vi "C(T) data viewer.vi"(0 "Cap Estimates":dbl[](array[numeric])=[1.269612045289484e-08, 1.3697308669126022e-08, 1.399985901178697e-08, 1.3777895246644411e-08, 1.3379717594157467e-08, 1.2501459178740452e-08, 1.1791524271713885e-08] format="%.2f", 1 "Temps":dbl[](array[numeric])=[26.0, 30.0, 34.0, 38.0, 42.0, 46.0, 50.0] format="%.2f", 2 "N Temps":i32=7, 5 "Resistance (Ohms)":dbl=100000.0 format="%.4e", 7 "Timing Control Parameters":T1={"N cycles for averaging"=300, "N points per measurement"=1000, "Measurment time interval"=2e-05} {"Measurment time interval" format="%.2e"}, 9 "waveforms":waveform(dbl)[](array[waveform])=[{"t0"=timestamp(3087922235.213 s since 1904-01-01), "dt"=1.9999999494757503e-05, "Y"=array[1000 elements]}, {"t0"=timestamp(3087922405.147 s since 1904-01-01), "dt"=1.9999999494757503e-05, "Y"=array[1000 elements]}, {"t0"=timestamp(3087922549.515 s since 1904-01-01), "dt"=1.9999999494757503e-05, "Y"=array[1000 elements]}, {"t0"=timestamp(3087922690.9379997 s since 1904-01-01), "dt"=1.9999999494757503e-05, "Y"=array[1000 elements]}, {"t0"=timestamp(3087922829.417 s since 1904-01-01), "dt"=1.9999999494757503e-05, "Y"=array[1000 elements]}, {"t0"=timestamp(3087922967.796 s since 1904-01-01), "dt"=1.9999999494757503e-05, "Y"=array[1000 elements]}, {"t0"=timestamp(3087923101.799 s since 1904-01-01), "dt"=1.9999999494757503e-05, "Y"=array[1000 elements]}], 11 "error in":errorcluster) -> (13 "no save out":bool, 15 "error out":errorcluster)   [LabVIEW 2016]
doc: "This vi allows the user to inspect the data before choosing to save it or not\n\nPaul K Dixon\nPhysics 350\nCSUSB Physics"
uses:
  globals/C(T) global variables.vi
panel:
  in  "Proceed no save":bool
  out "Resistance (Ohms)":dbl=100000.0 format="%.4e"
  out "Timing Control Parameters":T1={"N cycles for averaging"=300, "N points per measurement"=1000, "Measurment time interval"=2e-05} {"Measurment time interval" format="%.2e"}
  out "Number of Temperatures":i32=7
  out "Waveform":waveform(dbl)={"t0"=timestamp(3087922235.213 s since 1904-01-01), "dt"=1.9999999494757503e-05, "Y"=array[1000 elements]}
  out "Estimated Capacitance Value [nF]":i32(listbox) caption="choose the next state"
  out "Normalized decay versus time":waveform(dbl)(graph)={"t0"=timestamp(3087922235.213 s since 1904-01-01), "dt"=1.9999999494757503e-05, "Y"=array[1000 elements]}
  out "Cap versus Temp":cluster{"Temps":dbl[], dbl[]}[](graph)=[{"Temps"=[26.0, 30.0, 34.0, 38.0, 42.0, 46.0, 50.0], [12.69612045289484, 13.697308669126022, 13.99985901178697, 13.77789524664441, 13.379717594157466, 12.50145917874045, 11.791524271713884]}, {"Temps"=[26.0], [12.69612045289484]}] caption="Capacitance [nF] versus Temperature [Degrees C]"
  in  "Proceed":bool
  in  "Temperature to Display [C]":i32(listbox) caption="choose the next state"
  in  "Y Scale Mapping Mode":enum16{"Linear", "Logarithmic"}(ring)
  # "C(T) Data Viewer"
  # "General Parameters"
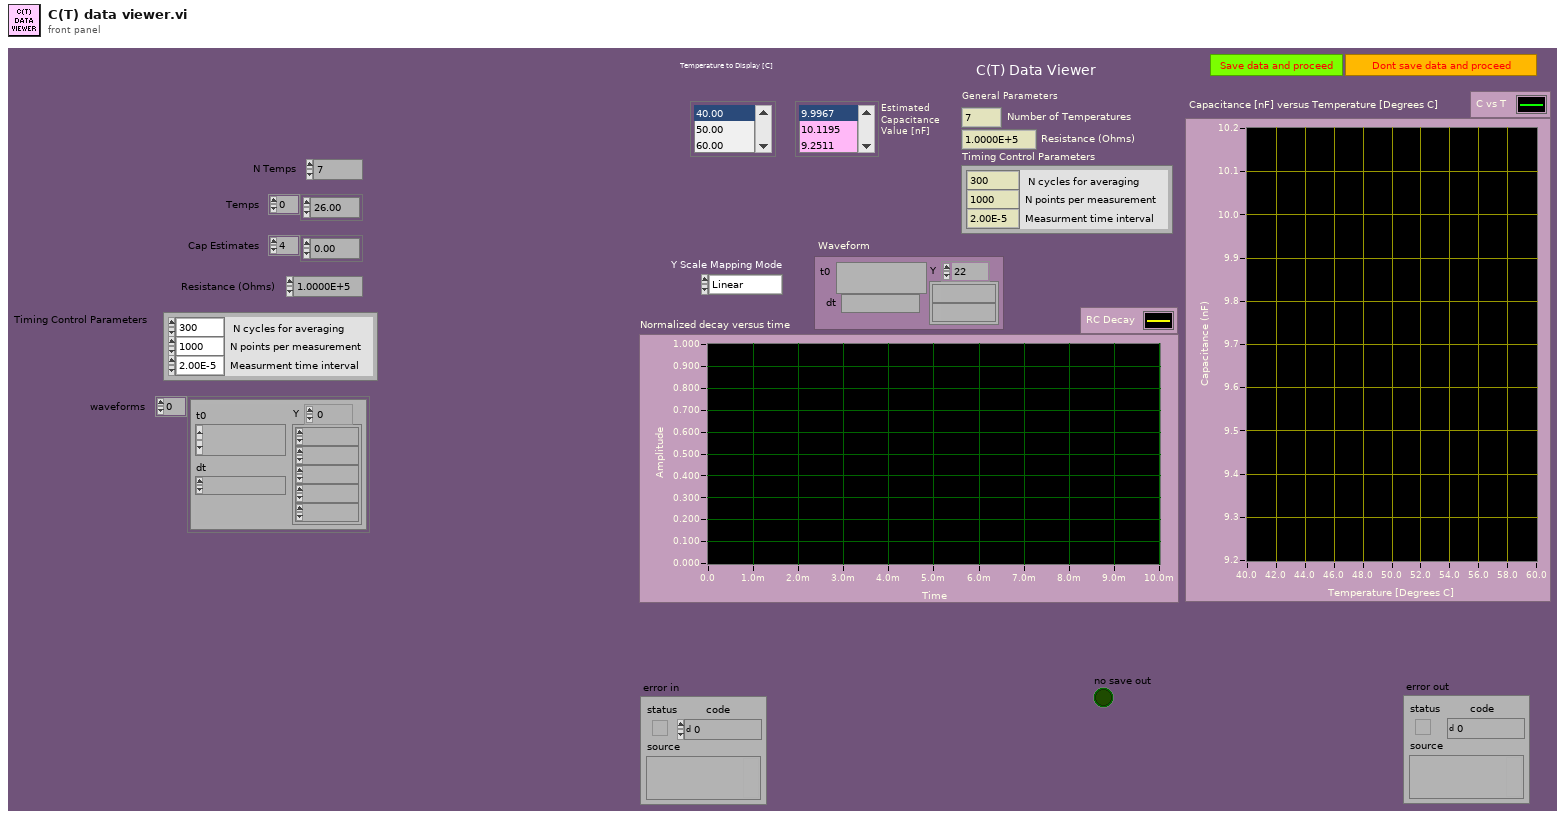
[diagram p1: front panel]
types:
  T1 = cluster{"N cycles for averaging":i32, "N points per measurement":i32, "Measurment time interval":dbl}
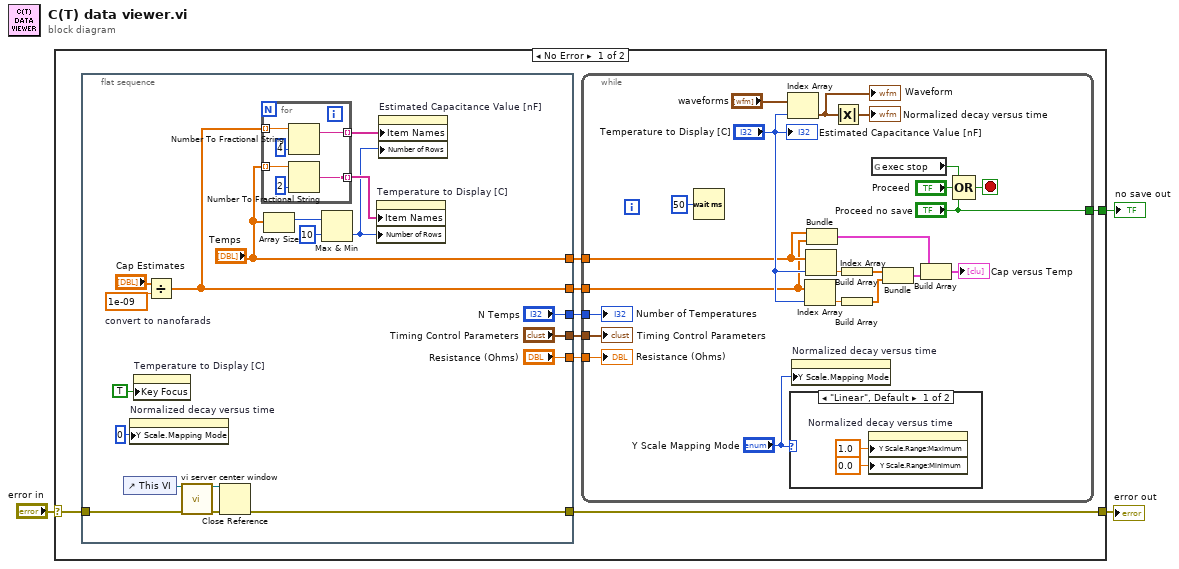
[diagram p0: block diagram]
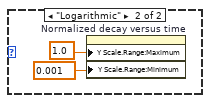
[diagram p2: hidden frame]
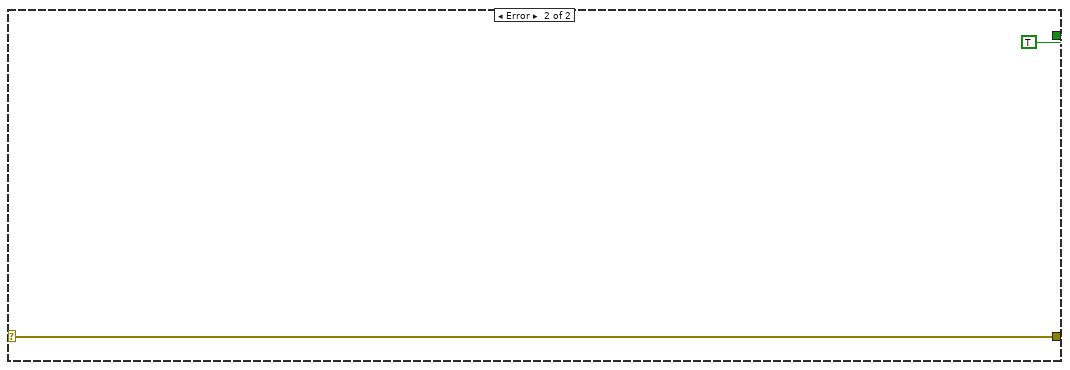
[diagram p3: hidden frame]
diagram:
  n1 = case shown="No Error" "error in" {
    selector: "error in" -> [w8 w64]
    tunnel: [w4 w64] -> w2
    tunnel: [w5 TRUE ("Proceed no save")] -> w1
    frame No Error {
      n2 = flat-sequence {
        tunnel: ["N Temps"] -> w11
        tunnel: ["Timing Control Parameters"] -> w10
        tunnel: ["Resistance (Ohms)"] -> w9
        tunnel: w8 -> [w20]
        tunnel: ["Temps"] -> w7
        tunnel: [w18] -> w6
        tunnel: [w16] -> w4
        frame #0 {
          w30 = 1e-09  # convert to nanofarads
          n3 = control-ref of="This VI"() -> (w14:refnum<vi>)
          n4 = property on="Normalized decay versus time" class="WFGraph (strict)"("Y Scale.Mapping Mode"=u8 0) -> ()  [unwired: 2 in, 2 out]
          n5 = property on="Temperature to Display [C]" class="LstBox (strict)"("Key Focus"=TRUE) -> ()  [unwired: 2 in, 2 out]
          n6 = Divide(x="Cap Estimates", y=w30) -> (x/y=w18:dbl[])
          n7 = call "vi server center window.vi"("VI ref in"=w14, "error in"=w20) -> ("VI ref out"=w15:refnum<vi>, "error out"=w17:errorcluster)  [unwired: 12 out]
          n8 = Close Reference(reference=w15, error in (no error)=w17) -> (error out=w16:errorcluster)
          n9 = for {
            tunnel: "Temps" -> [w36] mode=indexing
            tunnel: [w34] -> w26 mode=indexing
            tunnel: w18 -> [w32] mode=indexing
            tunnel: [w31] -> w21 mode=indexing
            n10 = Number To Fractional String(number=w32, precision (6)=i16 4) -> (F-format string=w31:string)  [unwired: 2 out]
            n11 = Number To Fractional String(number=w36, precision (6)=i16 2) -> (F-format string=w34:string)  [unwired: 2 out]
          }
          n12 = Array Size(array="Temps") -> (size(s)=w27:i32)
          n13 = Max & Min(x=w27, y=10) -> (min(x,y)=w22:i32)  [unwired: 1 out]
          n14 = property on="Temperature to Display [C]" class="LstBox (strict)"("Item Names"=w26, "Number of Rows"=w22) -> ()  [unwired: 2 in, 2 out]
          n15 = property on="Estimated Capacitance Value [nF]" class="LstBox (strict)"("Item Names"=w21, "Number of Rows"=w22) -> ()  [unwired: 2 in, 2 out]
        }
      }
      n16 = while {
        tunnel: w6 -> [w44]
        tunnel: w7 -> [w45]
        tunnel: w9 -> [w53]
        tunnel: w10 -> [w54]
        tunnel: w11 -> [w55]
        tunnel: ["Proceed no save"] -> w5
        stop <- w39 stop-if-true
        n17 = Wait (ms)(milliseconds to wait=u32 50) -> ()  [unwired: 1 out]
        n18 = Index Array(array="waveforms", index="Temperature to Display [C]") -> (element=w56:waveform(dbl))
        "Waveform" <- w56
        n19 = case shown="\"Linear\", Default" "Y Scale Mapping Mode" {
          frame "Linear", Default {
            n20 = property on="Normalized decay versus time" class="WFGraph (strict)"("Y Scale.Range:Maximum"=1.0, "Y Scale.Range:Minimum"=0.0) -> ()  [unwired: 2 in, 2 out]
          }
          frame "Logarithmic" {
            n21 = property on="Normalized decay versus time" class="WFGraph (strict)"("Y Scale.Range:Maximum"=1.0, "Y Scale.Range:Minimum"=0.001) -> ()  [unwired: 2 in, 2 out]
          }
        }
        n22 = property on="Normalized decay versus time" class="WFGraph (strict)"("Y Scale.Mapping Mode"="Y Scale Mapping Mode") -> ()  [unwired: 2 in, 2 out]
        n23 = Index Array(array=w44, index="Temperature to Display [C]") -> (element=w48:dbl)
        n24 = Index Array(array=w45, index="Temperature to Display [C]") -> (element=w49:dbl)
        n25 = Bundle("Temps"=w45, w44) -> (w43:cluster{"Temps":dbl[], dbl[]})  [unwired: 1 out]
        n26 = Absolute Value(x=w56) -> (abs(x)=→"Normalized decay versus time":waveform(dbl))
        n27 = Build Array(w49) -> (w46:dbl[])
        n28 = Build Array(w48) -> (w47:dbl[])
        n29 = global read "C(T) global variables.vi" "exec stop"() -> (w38:bool)
        n30 = Bundle(w46, w47) -> (w42:cluster{dbl[], dbl[]})  [unwired: 1 out]
        n31 = Build Array(w43, w42) -> (→"Cap versus Temp":cluster{"Temps":dbl[], dbl[]}[])
        n32 = Compound Arithmetic op=OR(w38, "Proceed", "Proceed no save") -> (w39:bool)
        "Number of Temperatures" <- w55
        "Timing Control Parameters" <- w54
        "Resistance (Ohms)" <- w53
        "Estimated Capacitance Value [nF]" <- "Temperature to Display [C]"
      }
    }
    frame Error {
    }
  }
  "error out" <- w2
  "no save out" <- w1
